vi "Main_pc.vi"() -> ()   [LabVIEW 2021]
panel:
  out "error out":errorcluster
  out "Duty cycle":dbl
  out "Angle":dbl
  in  "error in (no error)":errorcluster
  out "Boolean":bool
  in  "door programma":dbl
  in  "Pomp":bool
  out "Y":bool
  out "X":bool
  in  "Servo Y":dbl(slide) scale=0.0..180.0
  in  "Servo X":dbl(slide) scale=0.0..180.0
  in  "Manuele override":bool
  in  "?":bool
  out "Servo Y":dbl(knob) scale=0.0..180.0
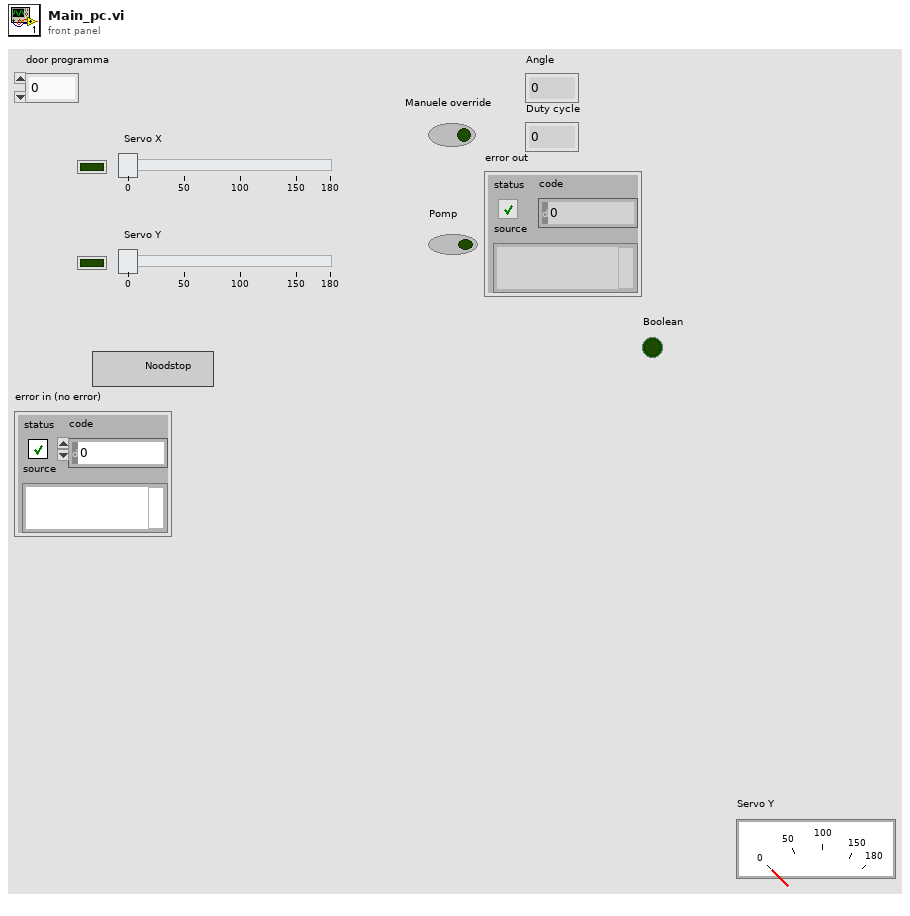
[diagram p1: front panel]
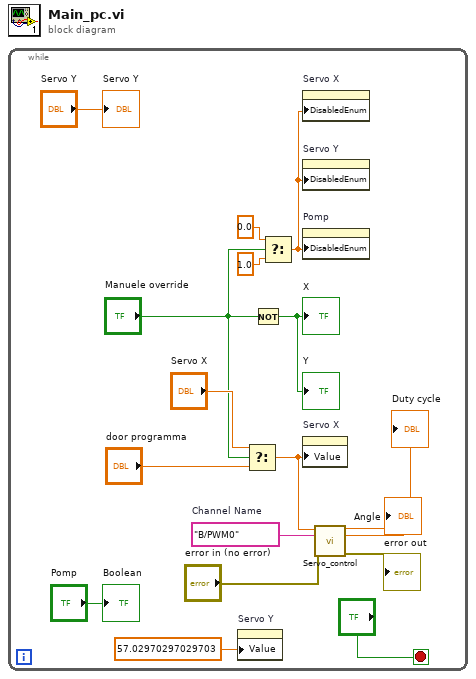
[diagram p0: block diagram]
diagram:
  n1 = while {
    stop <- "?" stop-if-true
    w5 = tag "B/PWM0"  # Channel Name
    n2 = property on="Servo Y" class="Slide (strict)"("Value"=57.02970297029703 ("Servo Y")) -> ()  [unwired: 2 in, 2 out]
    n3 = Select(t="Servo X", s="Manuele override", f="door programma") -> (s? t:f=w6:dbl)
    n4 = Not(x="Manuele override") -> (.not. x?=→"X" →"Y":bool)
    n5 = Select(t=0.0, s="Manuele override", f=1.0) -> (s? t:f=w13:dbl)
    n6 = property on="Servo X" class="Slide (strict)"("DisabledEnum"=w13) -> ()  [unwired: 2 in, 2 out]
    n7 = property on="Servo Y" class="Slide (strict)"("DisabledEnum"=w13) -> ()  [unwired: 2 in, 2 out]
    n8 = property on="Pomp" class="Bool (strict)"("DisabledEnum"=w13) -> ()  [unwired: 2 in, 2 out]
    n9 = property on="Servo X" class="Slide (strict)"("Value"=w6) -> ()  [unwired: 2 in, 2 out]
    n10 = call "Servo_control.vi"("Slide in"=w6, "Channel Name"=w5, "error in (no error)"="error in (no error)") -> ("Duty cycle"=→"Duty cycle":dbl, "Angle"=→"Angle":dbl, "error out"=→"error out":errorcluster)  [unwired: 10 in]
    "Servo Y" <- "Servo Y"
    "Boolean" <- "Pomp"
  }
